vi "Settings IO.vi"(7 "SettingsFileIO_Commands":T2, 8 "Error In":errorcluster, 10 "File Path (for scan specific settings)":path, 11 "Settings Array IN":T1[](array[typedef])) -> (0 "Error Out":errorcluster, 2 "Cancelled?":bool, 3 "Settings Array OUT":T1[](array[typedef]))   [LabVIEW 2012]
doc: "SciScan 1.2 160622"
uses:
  Settings IO_Commands.ctl
  Plugins/Macro Module/MacroGUI Module/Custom Controls and Typedefs/GFG Variable for IO.ctl
panel:
  out "Not found?":bool
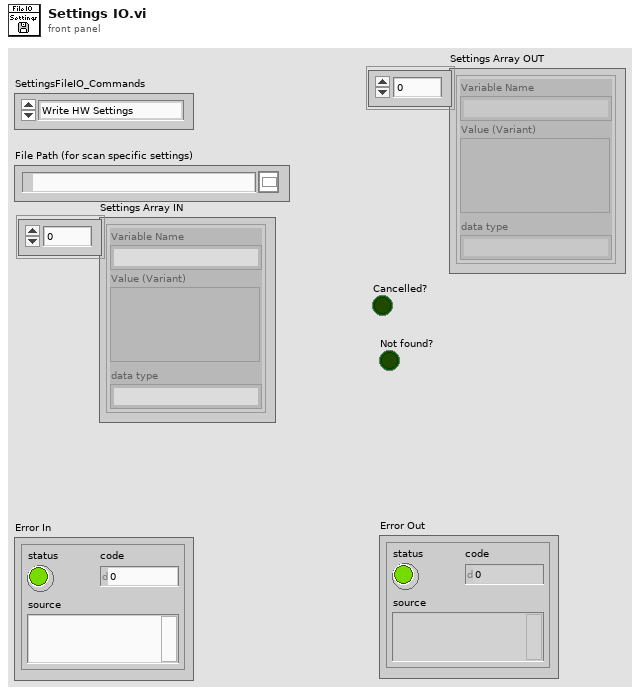
[diagram p1: front panel]
types:
  T1 = typedef "GFG Variable for IO.ctl" = cluster{"Variable Name":string, "Value (Variant)":variant, "data type":string}
  T2 = typedef "Settings IO_Commands.ctl" = enum16{"Write HW Settings", "Write Config Settings", "Read HW Settings", "Read Config Settings", "Write Line-Scan Settings", "Write Frame-Scan Settings", "Write Z-Stack Settings", "Read Line-Scan Settings", "Read Frame-Scan Settings", "Read Z-Stack Settings", "Read Fast-Z Settings", "Write Fast-Z Settings"}
  T3 = typedef "File Operation Status.ctl" = enum16{"Success", "File does not exist", "Cancelled by User", "Incorrect extension type"}
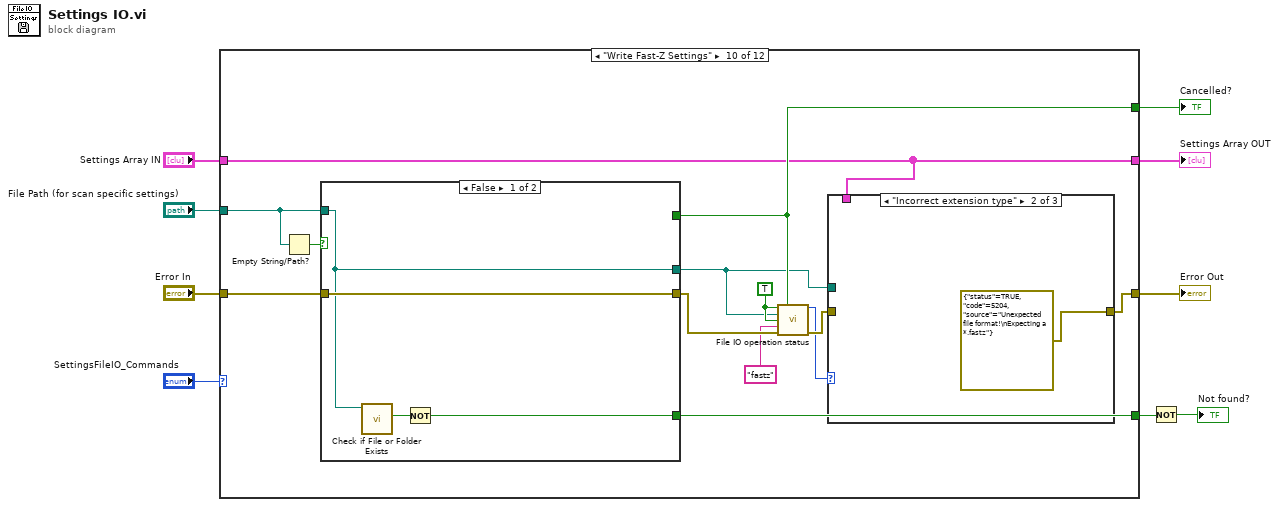
[diagram p0: block diagram]
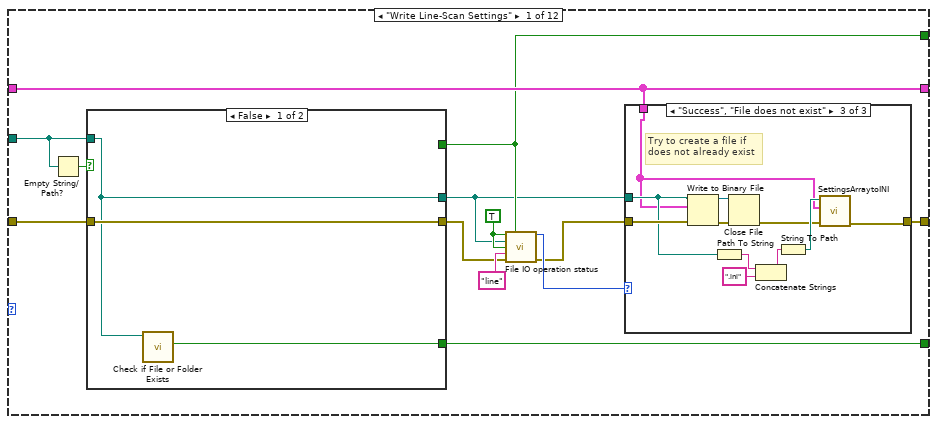
[diagram p2: hidden frame]
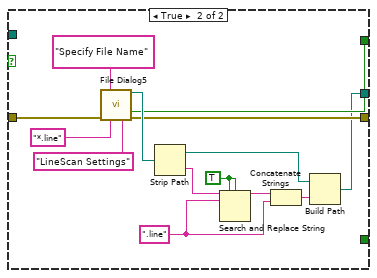
[diagram p3: hidden frame]
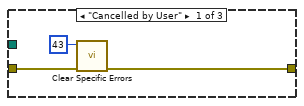
[diagram p4: hidden frame]
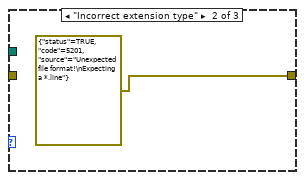
[diagram p5: hidden frame]
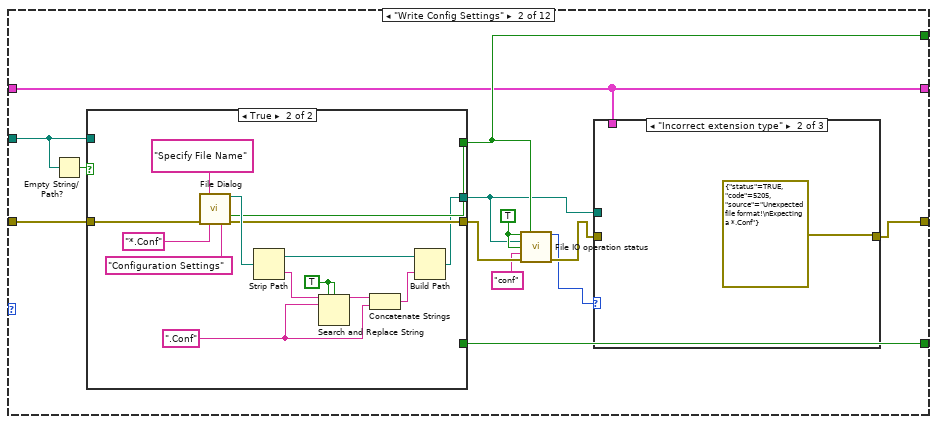
[diagram p6: hidden frame]
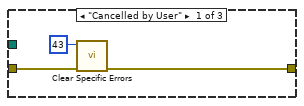
[diagram p7: hidden frame]
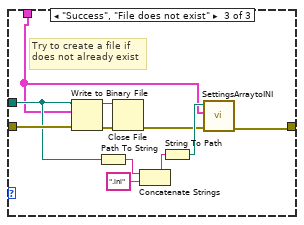
[diagram p8: hidden frame]
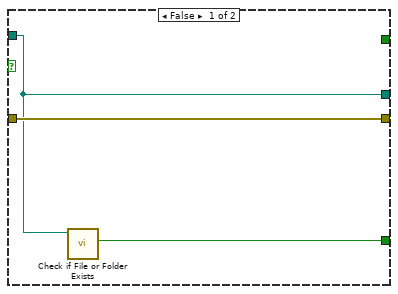
[diagram p9: hidden frame]
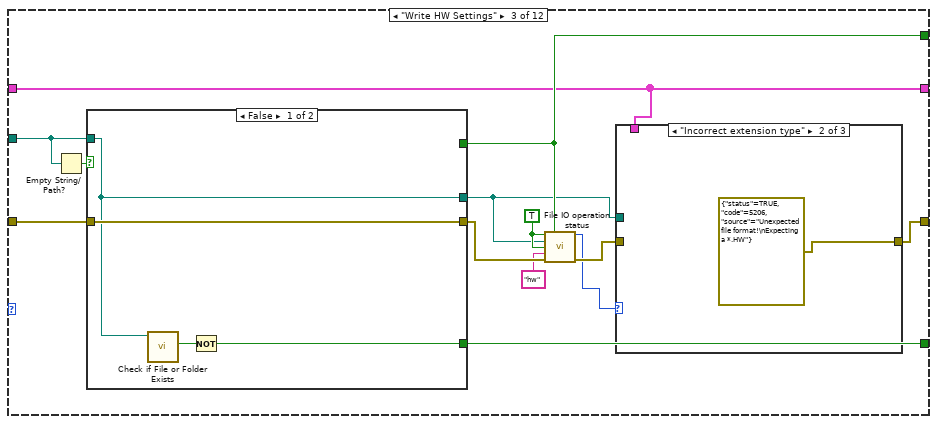
[diagram p10: hidden frame]
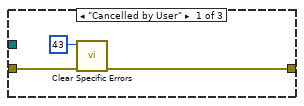
[diagram p11: hidden frame]
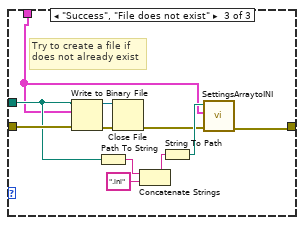
[diagram p12: hidden frame]
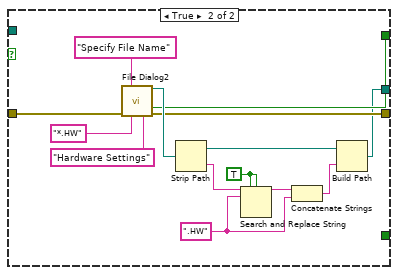
[diagram p13: hidden frame]
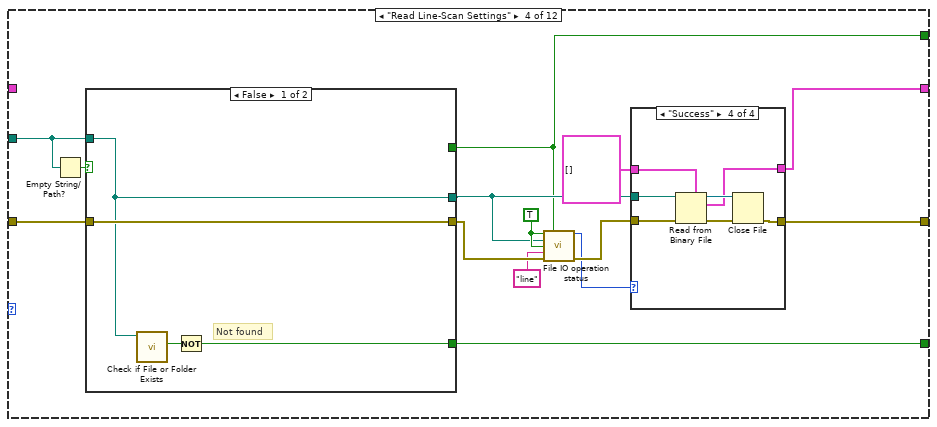
[diagram p14: hidden frame]
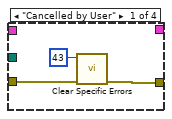
[diagram p15: hidden frame]
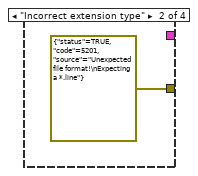
[diagram p16: hidden frame]
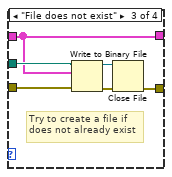
[diagram p17: hidden frame]
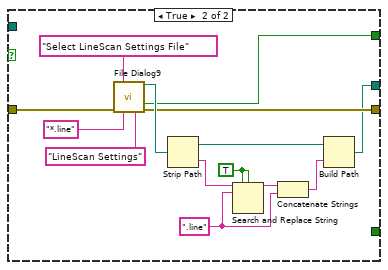
[diagram p18: hidden frame]
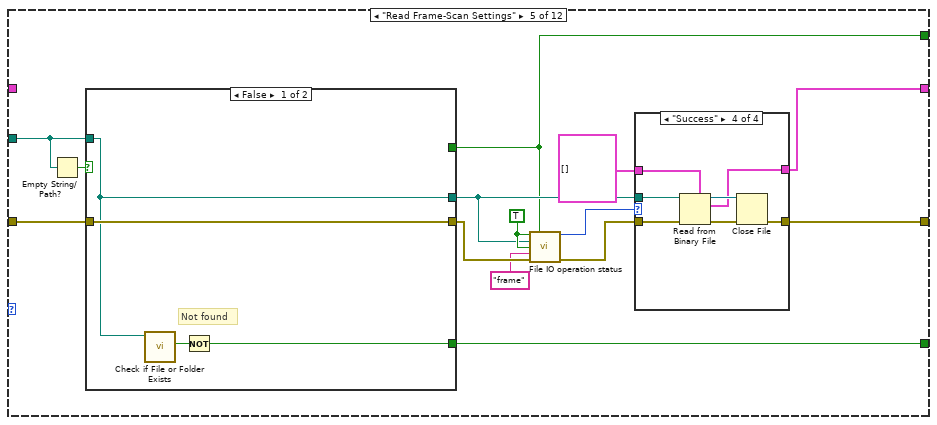
[diagram p19: hidden frame]
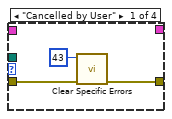
[diagram p20: hidden frame]
diagram:
  n1 = case shown="\"Write Fast-Z Settings\"" "SettingsFileIO_Commands" {
    tunnel: "Settings Array IN" -> [w22 w59 w104 _ _ _ _ w346 w391 w438 _ _]
    tunnel: [w12 w62 w105 w148 w196 w244 w296 w348 w393 w439 w483 w531] -> w7
    tunnel: [w22 w59 w104 w147 w198 w248 w293 w346 w391 w438 w481 w532] -> w6
    tunnel: [w21 w55 w100 w146 w200 w249 w298 w343 w392 w434 w482 w533] -> w5
    tunnel: "Error In" -> [w20 w67 w112 w159 w208 w257 w306 w354 w400 w446 w493 w541]
    tunnel: "File Path (for scan specific settings)" -> [w19 w66 w111 w157 w207 w255 w304 w353 w399 w445 w491 w540]
    tunnel: [w17 w64 w109 w156 w205 w254 w303 w351 w397 w443 w490 w538] -> w2
    frame "Write Line-Scan Settings" {
      w15 = TRUE
      n2 = Empty String/Path?(string/path=w19) -> (empty?=w18:bool)
      n3 = case shown="False" w18 {
        tunnel: [_ w31] -> w12
        tunnel: w20 -> [w25 w28]
        tunnel: [w25 w27] -> w13
        tunnel: w19 -> [w24 _]
        tunnel: [w24 w26] -> w10
        tunnel: [w23 _] -> w17
        frame False {
          n4 = call <vilib>:"Check if File or Folder Exists.vi"("path"=w24) -> ("file or folder exists?"=w23:bool)  [unwired: 8 in, 2 out]
        }
        frame True {
          w32 = ".line" ("pattern (all files)")
          w37 = TRUE ("replace all? (F)")
          n5 = call "File Dialog5"("prompt"="Specify File Name", "error in"=w28, "pattern (all files)"="*.line", "pattern label"="LineScan Settings") -> ("selected path"=w34:path, "cancelled"=w31:bool, "error out"=w27:errorcluster)  [unwired: 8 in, 1 out]
          n6 = Strip Path(path=w34) -> (stripped path=w29:path, name=w36:string)
          n7 = Search and Replace String(replace all?=w37, case sensitive?=w37, input string=w36, search string=w32) -> (result string=w35:string)  [unwired: 4 in, 3 out]
          n8 = Concatenate Strings(w35, w32) -> (w30:string)
          n9 = Build Path(base path=w29, name or relative path=w30) -> (appended path=w26:path)
        }
      }
      n10 = call "File IO operation status.vi"("check if valid path (Specify File Path)"=w15, "Cancelled by User? (status from a previous dialog)"=w12, "File Path"=w10, "check if valid extension (Specify Extension Type)"=w15, "expected extension type"="line" ("string"), "error in (no error)"=w13) -> ("File Operation Status"=w14:T3, "error out"=w11:errorcluster)  [unwired: 8 in]
      n11 = case shown="\"Success\", \"File does not exist\"" w14 {
        tunnel: w22 -> [_ _ w44]
        tunnel: [w40 errorcluster {"status"=TRUE, "code"=5201, "source"="Unexpected file format!\nExpecting a *.line"} ("error constant") w47] -> w21
        tunnel: w11 -> [w41 _ w52]
        tunnel: w10 -> [_ _ w45]
        frame "Cancelled by User" {
          n12 = call "Clear Specific Errors.vi"("Error In"=w41, "Error number In"=43) -> ("Error Out"=w40:errorcluster)  [unwired: 8 in, 1 out]
        }
        frame "Incorrect extension type" {
        }
        frame "Success", "File does not exist" {
          # "Try to create a file if \ndoes not already exist"
          n13 = Write to Binary File(file (use dialog)=w45, data=w44, error in=w52) -> (refnum out=w54:refnum<file>, error out=w53:errorcluster)  [unwired: 3 in, 1 out]
          n14 = Path To String(path=w45) -> (string=w48:string)
          n15 = Close File(refnum=w54, error in=w53) -> (error out=w46:errorcluster)  [unwired: 1 out]
          n16 = Concatenate Strings(w48, ".ini" ("string")) -> (w50:string)
          n17 = String To Path(string=w50) -> (path=w51:path)
          n18 = call "SettingsArraytoINI.vi"("error in (no error)"=w46, "Settings Array IN"=w44, "Path"=w51) -> ("error out"=w47:errorcluster)  [unwired: 8 in]
        }
      }
    }
    frame "Write Config Settings" {
      w63 = TRUE
      n19 = Empty String/Path?(string/path=w66) -> (empty?=w65:bool)
      n20 = case shown="True" w65 {
        tunnel: [_ w91] -> w62
        tunnel: w67 -> [w85 w88]
        tunnel: [w85 w87] -> w61
        tunnel: w66 -> [w84 _]
        tunnel: [w84 w86] -> w58
        tunnel: [w83 _] -> w64
        frame False {
          n21 = call <vilib>:"Check if File or Folder Exists.vi"("path"=w84) -> ("file or folder exists?"=w83:bool)  [unwired: 8 in, 2 out]
        }
        frame True {
          w92 = ".Conf" ("pattern (all files)")
          w97 = TRUE ("replace all? (F)")
          n22 = call "File Dialog"("prompt"="Specify File Name", "error in"=w88, "pattern (all files)"="*.Conf", "pattern label"="Configuration Settings") -> ("selected path"=w94:path, "cancelled"=w91:bool, "error out"=w87:errorcluster)  [unwired: 8 in, 1 out]
          n23 = Strip Path(path=w94) -> (stripped path=w89:path, name=w96:string)
          n24 = Search and Replace String(replace all?=w97, case sensitive?=w97, input string=w96, search string=w92) -> (result string=w95:string)  [unwired: 4 in, 3 out]
          n25 = Concatenate Strings(w95, w92) -> (w90:string)
          n26 = Build Path(base path=w89, name or relative path=w90) -> (appended path=w86:path)
        }
      }
      n27 = call "File IO operation status.vi"("check if valid path (Specify File Path)"=w63, "Cancelled by User? (status from a previous dialog)"=w62, "File Path"=w58, "check if valid extension (Specify Extension Type)"=w63, "expected extension type"="conf" ("string"), "error in (no error)"=w61) -> ("File Operation Status"=w56:T3, "error out"=w57:errorcluster)  [unwired: 8 in]
      n28 = case shown="\"Incorrect extension type\"" w56 {
        tunnel: w59 -> [_ _ w72]
        tunnel: [w68 errorcluster {"status"=TRUE, "code"=5205, "source"="Unexpected file format!\nExpecting a *.Conf"} ("error constant") w75] -> w55
        tunnel: w57 -> [w69 _ w80]
        tunnel: w58 -> [_ _ w73]
        frame "Cancelled by User" {
          n29 = call "Clear Specific Errors.vi"("Error In"=w69, "Error number In"=43) -> ("Error Out"=w68:errorcluster)  [unwired: 8 in, 1 out]
        }
        frame "Incorrect extension type" {
        }
        frame "Success", "File does not exist" {
          # "Try to create a file if \ndoes not already exist"
          n30 = Write to Binary File(file (use dialog)=w73, data=w72, error in=w80) -> (refnum out=w82:refnum<file>, error out=w81:errorcluster)  [unwired: 3 in, 1 out]
          n31 = Path To String(path=w73) -> (string=w76:string)
          n32 = Close File(refnum=w82, error in=w81) -> (error out=w74:errorcluster)  [unwired: 1 out]
          n33 = Concatenate Strings(w76, ".ini" ("string")) -> (w78:string)
          n34 = String To Path(string=w78) -> (path=w79:path)
          n35 = call "SettingsArraytoINI.vi"("error in (no error)"=w74, "Settings Array IN"=w72, "Path"=w79) -> ("error out"=w75:errorcluster)  [unwired: 8 in]
        }
      }
    }
    frame "Write HW Settings" {
      w108 = TRUE
      n36 = Empty String/Path?(string/path=w111) -> (empty?=w110:bool)
      n37 = case shown="False" w110 {
        tunnel: [_ w137] -> w105
        tunnel: w112 -> [w131 w134]
        tunnel: [w131 w133] -> w107
        tunnel: w111 -> [w129 _]
        tunnel: [w129 w132] -> w103
        tunnel: [w128 _] -> w109
        frame False {
          n38 = call <vilib>:"Check if File or Folder Exists.vi"("path"=w129) -> ("file or folder exists?"=w130:bool)  [unwired: 8 in, 2 out]
          n39 = Not(x=w130) -> (.not. x?=w128:bool)
        }
        frame True {
          w138 = ".HW" ("pattern (all files)")
          w143 = TRUE ("replace all? (F)")
          n40 = call "File Dialog2"("prompt"="Specify File Name", "error in"=w134, "pattern (all files)"="*.HW", "pattern label"="Hardware Settings") -> ("selected path"=w140:path, "cancelled"=w137:bool, "error out"=w133:errorcluster)  [unwired: 8 in, 1 out]
          n41 = Strip Path(path=w140) -> (stripped path=w135:path, name=w142:string)
          n42 = Search and Replace String(replace all?=w143, case sensitive?=w143, input string=w142, search string=w138) -> (result string=w141:string)  [unwired: 4 in, 3 out]
          n43 = Concatenate Strings(w141, w138) -> (w136:string)
          n44 = Build Path(base path=w135, name or relative path=w136) -> (appended path=w132:path)
        }
      }
      n45 = call "File IO operation status.vi"("check if valid path (Specify File Path)"=w108, "Cancelled by User? (status from a previous dialog)"=w105, "File Path"=w103, "check if valid extension (Specify Extension Type)"=w108, "expected extension type"="hw" ("string"), "error in (no error)"=w107) -> ("File Operation Status"=w101:T3, "error out"=w102:errorcluster)  [unwired: 8 in]
      n46 = case shown="\"Incorrect extension type\"" w101 {
        tunnel: w104 -> [_ _ w117]
        tunnel: [w113 errorcluster {"status"=TRUE, "code"=5206, "source"="Unexpected file format!\nExpecting a *.HW"} ("error constant") w120] -> w100
        tunnel: w102 -> [w114 _ w125]
        tunnel: w103 -> [_ _ w118]
        frame "Cancelled by User" {
          n47 = call "Clear Specific Errors.vi"("Error In"=w114, "Error number In"=43) -> ("Error Out"=w113:errorcluster)  [unwired: 8 in, 1 out]
        }
        frame "Incorrect extension type" {
        }
        frame "Success", "File does not exist" {
          # "Try to create a file if \ndoes not already exist"
          n48 = Write to Binary File(file (use dialog)=w118, data=w117, error in=w125) -> (refnum out=w127:refnum<file>, error out=w126:errorcluster)  [unwired: 3 in, 1 out]
          n49 = Path To String(path=w118) -> (string=w121:string)
          n50 = Close File(refnum=w127, error in=w126) -> (error out=w119:errorcluster)  [unwired: 1 out]
          n51 = Concatenate Strings(w121, ".ini" ("string")) -> (w123:string)
          n52 = String To Path(string=w123) -> (path=w124:path)
          n53 = call "SettingsArraytoINI.vi"("error in (no error)"=w119, "Settings Array IN"=w117, "Path"=w124) -> ("error out"=w120:errorcluster)  [unwired: 8 in]
        }
      }
    }
    frame "Read Line-Scan Settings" {
      w152 = TRUE
      n54 = Empty String/Path?(string/path=w157) -> (empty?=w158:bool)
      n55 = case shown="False" w158 {
        tunnel: w159 -> [w180 w184]
        tunnel: [w180 w183] -> w151
        tunnel: [w178 w182] -> w149
        tunnel: [_ w181] -> w148
        tunnel: w157 -> [w178 _]
        tunnel: [w177 _] -> w156
        frame False {
          # "Not found"
          n56 = call <vilib>:"Check if File or Folder Exists.vi"("path"=w178) -> ("file or folder exists?"=w179:bool)  [unwired: 8 in, 2 out]
          n57 = Not(x=w179) -> (.not. x?=w177:bool)
        }
        frame True {
          w185 = ".line" ("pattern (all files)")
          w192 = TRUE ("replace all? (F)")
          n58 = call "File Dialog9"("prompt"="Select LineScan Settings File", "error in"=w184, "pattern (all files)"="*.line", "pattern label"="LineScan Settings") -> ("selected path"=w187:path, "cancelled"=w181:bool, "error out"=w183:errorcluster)  [unwired: 8 in, 1 out]
          n59 = Strip Path(path=w187) -> (stripped path=w189:path, name=w191:string)
          n60 = Search and Replace String(replace all?=w192, case sensitive?=w192, input string=w191, search string=w185) -> (result string=w190:string)  [unwired: 4 in, 3 out]
          n61 = Concatenate Strings(w190, w185) -> (w188:string)
          n62 = Build Path(base path=w189, name or relative path=w188) -> (appended path=w182:path)
        }
      }
      n63 = call "File IO operation status.vi"("check if valid path (Specify File Path)"=w152, "Cancelled by User? (status from a previous dialog)"=w148, "File Path"=w149, "check if valid extension (Specify Extension Type)"=w152, "expected extension type"="line" ("string"), "error in (no error)"=w151) -> ("File Operation Status"=w153:T3, "error out"=w154:errorcluster)  [unwired: 8 in]
      n64 = case shown="\"Success\"" w153 {
        tunnel: T1[] [] ("Settings Array IN") -> [_ _ w164 w172]
        tunnel: [w160 errorcluster {"status"=TRUE, "code"=5201, "source"="Unexpected file format!\nExpecting a *.line"} ("error constant") w166 w173] -> w146
        tunnel: w154 -> [w161 _ w167 w174]
        tunnel: w149 -> [_ _ w165 w170]
        tunnel: [_ _ w164 w171] -> w147
        frame "Cancelled by User" {
          n65 = call "Clear Specific Errors.vi"("Error In"=w161, "Error number In"=43) -> ("Error Out"=w160:errorcluster)  [unwired: 8 in, 1 out]
        }
        frame "Incorrect extension type" {
        }
        frame "File does not exist" {
          # "Try to create a file if \ndoes not already exist"
          n66 = Write to Binary File(file (use dialog)=w165, data=w164, error in=w167) -> (refnum out=w169:refnum<file>, error out=w168:errorcluster)  [unwired: 3 in, 1 out]
          n67 = Close File(refnum=w169, error in=w168) -> (error out=w166:errorcluster)  [unwired: 1 out]
        }
        frame "Success" {
          n68 = Read from Binary File(5:w172, 8:w174, 11:w170) -> (0:w176:errorcluster, 2:w171:T1[], 3:w175:refnum<file>)  [unwired: 3 in, 1 out]
          n69 = Close File(refnum=w175, error in=w176) -> (error out=w173:errorcluster)  [unwired: 1 out]
        }
      }
    }
    frame "Read Frame-Scan Settings" {
      w201 = TRUE
      n70 = Empty String/Path?(string/path=w207) -> (empty?=w206:bool)
      n71 = case shown="False" w206 {
        tunnel: w208 -> [w229 w233]
        tunnel: [w229 w232] -> w199
        tunnel: [w227 w231] -> w197
        tunnel: [_ w230] -> w196
        tunnel: w207 -> [w227 _]
        tunnel: [w226 _] -> w205
        frame False {
          # "Not found"
          n72 = call <vilib>:"Check if File or Folder Exists.vi"("path"=w227) -> ("file or folder exists?"=w228:bool)  [unwired: 8 in, 2 out]
          n73 = Not(x=w228) -> (.not. x?=w226:bool)
        }
        frame True {
          w234 = ".frame" ("pattern (all files)")
          w241 = TRUE ("replace all? (F)")
          n74 = call "File Dialog10"("prompt"="Select FrameScan Settings File", "error in"=w233, "pattern (all files)"="*.frame", "pattern label"="FrameScan Settings") -> ("selected path"=w236:path, "cancelled"=w230:bool, "error out"=w232:errorcluster)  [unwired: 8 in, 1 out]
          n75 = Strip Path(path=w236) -> (stripped path=w238:path, name=w240:string)
          n76 = Search and Replace String(replace all?=w241, case sensitive?=w241, input string=w240, search string=w234) -> (result string=w239:string)  [unwired: 4 in, 3 out]
          n77 = Concatenate Strings(w239, w234) -> (w237:string)
          n78 = Build Path(base path=w238, name or relative path=w237) -> (appended path=w231:path)
        }
      }
      n79 = call "File IO operation status.vi"("check if valid path (Specify File Path)"=w201, "Cancelled by User? (status from a previous dialog)"=w196, "File Path"=w197, "check if valid extension (Specify Extension Type)"=w201, "expected extension type"="frame" ("string"), "error in (no error)"=w199) -> ("File Operation Status"=w202:T3, "error out"=w203:errorcluster)  [unwired: 8 in]
      n80 = case shown="\"Success\"" w202 {
        tunnel: T1[] [] ("Settings Array IN") -> [_ _ w213 w221]
        tunnel: [w209 errorcluster {"status"=TRUE, "code"=5202, "source"="Unexpected file format!\nExpecting a *.frame"} ("error constant") w215 w222] -> w200
        tunnel: w203 -> [w210 _ w216 w223]
        tunnel: w197 -> [_ _ w214 w219]
        tunnel: [_ _ w213 w220] -> w198
        frame "Cancelled by User" {
          n81 = call "Clear Specific Errors.vi"("Error In"=w210, "Error number In"=43) -> ("Error Out"=w209:errorcluster)  [unwired: 8 in, 1 out]
        }
        frame "Incorrect extension type" {
        }
        frame "File does not exist" {
          # "Try to create a file if \ndoes not already exist"
          n82 = Write to Binary File(file (use dialog)=w214, data=w213, error in=w216) -> (refnum out=w218:refnum<file>, error out=w217:errorcluster)  [unwired: 3 in, 1 out]
          n83 = Close File(refnum=w218, error in=w217) -> (error out=w215:errorcluster)  [unwired: 1 out]
        }
        frame "Success" {
          n84 = Read from Binary File(5:w221, 8:w223, 11:w219) -> (0:w225:errorcluster, 2:w220:T1[], 3:w224:refnum<file>)  [unwired: 3 in, 1 out]
          n85 = Close File(refnum=w224, error in=w225) -> (error out=w222:errorcluster)  [unwired: 1 out]
        }
      }
    }
    frame "Read Z-Stack Settings" {
      w250 = TRUE
      n86 = Empty String/Path?(string/path=w255) -> (empty?=w256:bool)
      n87 = case shown="True" w256 {
        tunnel: w257 -> [w278 w282]
        tunnel: [w278 w281] -> w247
        tunnel: [w276 w280] -> w246
        tunnel: [_ w279] -> w244
        tunnel: w255 -> [w276 _]
        tunnel: [w275 _] -> w254
        frame False {
          # "Not found"
          n88 = call <vilib>:"Check if File or Folder Exists.vi"("path"=w276) -> ("file or folder exists?"=w277:bool)  [unwired: 8 in, 2 out]
          n89 = Not(x=w277) -> (.not. x?=w275:bool)
        }
        frame True {
          w283 = ".zstack" ("pattern (all files)")
          w290 = TRUE ("replace all? (F)")
          n90 = call "File Dialog11"("prompt"="Select ZStack Settings File", "error in"=w282, "pattern (all files)"="*.zstack", "pattern label"="Z-Stack Settings") -> ("selected path"=w285:path, "cancelled"=w279:bool, "error out"=w281:errorcluster)  [unwired: 8 in, 1 out]
          n91 = Strip Path(path=w285) -> (stripped path=w287:path, name=w289:string)
          n92 = Search and Replace String(replace all?=w290, case sensitive?=w290, input string=w289, search string=w283) -> (result string=w288:string)  [unwired: 4 in, 3 out]
          n93 = Concatenate Strings(w288, w283) -> (w286:string)
          n94 = Build Path(base path=w287, name or relative path=w286) -> (appended path=w280:path)
        }
      }
      n95 = call "File IO operation status.vi"("check if valid path (Specify File Path)"=w250, "Cancelled by User? (status from a previous dialog)"=w244, "File Path"=w246, "check if valid extension (Specify Extension Type)"=w250, "expected extension type"="zstack" ("string"), "error in (no error)"=w247) -> ("File Operation Status"=w251:T3, "error out"=w252:errorcluster)  [unwired: 8 in]
      n96 = case shown="\"File does not exist\"" w251 {
        tunnel: T1[] [] ("Settings Array IN") -> [_ _ w262 w271]
        tunnel: [w258 errorcluster {"status"=TRUE, "code"=5203, "source"="Unexpected file format!\nExpecting a *.zstack"} ("error constant") w264 w268] -> w249
        tunnel: w252 -> [w259 _ w265 w272]
        tunnel: w246 -> [_ _ w263 w269]
        tunnel: [_ _ w262 w270] -> w248
        frame "Cancelled by User" {
          n97 = call "Clear Specific Errors.vi"("Error In"=w259, "Error number In"=43) -> ("Error Out"=w258:errorcluster)  [unwired: 8 in, 1 out]
        }
        frame "Incorrect extension type" {
        }
        frame "File does not exist" {
          # "Try to create a file if \ndoes not already exist"
          n98 = Write to Binary File(file (use dialog)=w263, data=w262, error in=w265) -> (refnum out=w267:refnum<file>, error out=w266:errorcluster)  [unwired: 3 in, 1 out]
          n99 = Close File(refnum=w267, error in=w266) -> (error out=w264:errorcluster)  [unwired: 1 out]
        }
        frame "Success" {
          n100 = Read from Binary File(5:w271, 8:w272, 11:w269) -> (0:w274:errorcluster, 2:w270:T1[], 3:w273:refnum<file>)  [unwired: 3 in, 1 out]
          n101 = Close File(refnum=w273, error in=w274) -> (error out=w268:errorcluster)  [unwired: 1 out]
        }
      }
    }
    frame "Read Fast-Z Settings" {
      w299 = TRUE
      n102 = Empty String/Path?(string/path=w304) -> (empty?=w305:bool)
      n103 = case shown="False" w305 {
        tunnel: w306 -> [w327 w331]
        tunnel: [w327 w330] -> w297
        tunnel: [w325 w329] -> w295
        tunnel: [_ w328] -> w296
        tunnel: w304 -> [w325 _]
        tunnel: [w324 _] -> w303
        frame False {
          # "Not found"
          n104 = call <vilib>:"Check if File or Folder Exists.vi"("path"=w325) -> ("file or folder exists?"=w326:bool)  [unwired: 8 in, 2 out]
          n105 = Not(x=w326) -> (.not. x?=w324:bool)
        }
        frame True {
          w332 = ".fastz" ("pattern (all files)")
          w339 = TRUE ("replace all? (F)")
          n106 = call "File Dialog6"("prompt"="Select Fast-Z Settings File", "error in"=w331, "pattern (all files)"="*.fastz", "pattern label"="Fast-Z Settings") -> ("selected path"=w334:path, "cancelled"=w328:bool, "error out"=w330:errorcluster)  [unwired: 8 in, 1 out]
          n107 = Strip Path(path=w334) -> (stripped path=w336:path, name=w338:string)
          n108 = Search and Replace String(replace all?=w339, case sensitive?=w339, input string=w338, search string=w332) -> (result string=w337:string)  [unwired: 4 in, 3 out]
          n109 = Concatenate Strings(w337, w332) -> (w335:string)
          n110 = Build Path(base path=w336, name or relative path=w335) -> (appended path=w329:path)
        }
      }
      n111 = call "File IO operation status.vi"("check if valid path (Specify File Path)"=w299, "Cancelled by User? (status from a previous dialog)"=w296, "File Path"=w295, "check if valid extension (Specify Extension Type)"=w299, "expected extension type"="fastz" ("string"), "error in (no error)"=w297) -> ("File Operation Status"=w300:T3, "error out"=w301:errorcluster)  [unwired: 8 in]
      n112 = case shown="\"Success\"" w300 {
        tunnel: T1[] [] ("Settings Array IN") -> [_ _ w311 w319]
        tunnel: [w307 errorcluster {"status"=TRUE, "code"=5204, "source"="Unexpected file format!\nExpecting a *.fastz"} ("error constant") w313 w320] -> w298
        tunnel: w301 -> [w308 _ w314 w321]
        tunnel: w295 -> [_ _ w312 w317]
        tunnel: [_ _ w311 w318] -> w293
        frame "Cancelled by User" {
          n113 = call "Clear Specific Errors.vi"("Error In"=w308, "Error number In"=43) -> ("Error Out"=w307:errorcluster)  [unwired: 8 in, 1 out]
        }
        frame "Incorrect extension type" {
        }
        frame "File does not exist" {
          # "Try to create a file if \ndoes not already exist"
          n114 = Write to Binary File(file (use dialog)=w312, data=w311, error in=w314) -> (refnum out=w316:refnum<file>, error out=w315:errorcluster)  [unwired: 3 in, 1 out]
          n115 = Close File(refnum=w316, error in=w315) -> (error out=w313:errorcluster)  [unwired: 1 out]
        }
        frame "Success" {
          n116 = Read from Binary File(5:w319, 8:w321, 11:w317) -> (0:w323:errorcluster, 2:w318:T1[], 3:w322:refnum<file>)  [unwired: 3 in, 1 out]
          n117 = Close File(refnum=w322, error in=w323) -> (error out=w320:errorcluster)  [unwired: 1 out]
        }
      }
    }
    frame "Write Frame-Scan Settings" {
      w350 = TRUE
      n118 = Empty String/Path?(string/path=w353) -> (empty?=w352:bool)
      n119 = case shown="False" w352 {
        tunnel: [_ w379] -> w348
        tunnel: w354 -> [w373 w376]
        tunnel: [w373 w375] -> w349
        tunnel: w353 -> [w371 _]
        tunnel: [w371 w374] -> w344
        tunnel: [w370 _] -> w351
        frame False {
          n120 = call <vilib>:"Check if File or Folder Exists.vi"("path"=w371) -> ("file or folder exists?"=w372:bool)  [unwired: 8 in, 2 out]
          n121 = Not(x=w372) -> (.not. x?=w370:bool)
        }
        frame True {
          w380 = ".frame" ("pattern (all files)")
          w385 = TRUE ("replace all? (F)")
          n122 = call "File Dialog7"("prompt"="Specify File Name", "error in"=w376, "pattern (all files)"="*.frame", "pattern label"="FrameScan Settings") -> ("selected path"=w382:path, "cancelled"=w379:bool, "error out"=w375:errorcluster)  [unwired: 8 in, 1 out]
          n123 = Strip Path(path=w382) -> (stripped path=w377:path, name=w384:string)
          n124 = Search and Replace String(replace all?=w385, case sensitive?=w385, input string=w384, search string=w380) -> (result string=w383:string)  [unwired: 4 in, 3 out]
          n125 = Concatenate Strings(w383, w380) -> (w378:string)
          n126 = Build Path(base path=w377, name or relative path=w378) -> (appended path=w374:path)
        }
      }
      n127 = call "File IO operation status.vi"("check if valid path (Specify File Path)"=w350, "Cancelled by User? (status from a previous dialog)"=w348, "File Path"=w344, "check if valid extension (Specify Extension Type)"=w350, "expected extension type"="frame" ("string"), "error in (no error)"=w349) -> ("File Operation Status"=w342:T3, "error out"=w345:errorcluster)  [unwired: 8 in]
      n128 = case shown="\"Incorrect extension type\"" w342 {
        tunnel: w346 -> [_ _ w359]
        tunnel: [w355 errorcluster {"status"=TRUE, "code"=5202, "source"="Unexpected file format!\nExpecting a *.frame"} ("error constant") w362] -> w343
        tunnel: w345 -> [w356 _ w367]
        tunnel: w344 -> [_ _ w360]
        frame "Cancelled by User" {
          n129 = call "Clear Specific Errors.vi"("Error In"=w356, "Error number In"=43) -> ("Error Out"=w355:errorcluster)  [unwired: 8 in, 1 out]
        }
        frame "Incorrect extension type" {
        }
        frame "Success", "File does not exist" {
          # "Try to create a file if \ndoes not already exist"
          n130 = Write to Binary File(file (use dialog)=w360, data=w359, error in=w367) -> (refnum out=w369:refnum<file>, error out=w368:errorcluster)  [unwired: 3 in, 1 out]
          n131 = Path To String(path=w360) -> (string=w363:string)
          n132 = Close File(refnum=w369, error in=w368) -> (error out=w361:errorcluster)  [unwired: 1 out]
          n133 = Concatenate Strings(w363, ".ini" ("string")) -> (w365:string)
          n134 = String To Path(string=w365) -> (path=w366:path)
          n135 = call "SettingsArraytoINI.vi"("error in (no error)"=w361, "Settings Array IN"=w359, "Path"=w366) -> ("error out"=w362:errorcluster)  [unwired: 8 in]
        }
      }
    }
    frame "Write Z-Stack Settings" {
      w396 = TRUE
      n136 = Empty String/Path?(string/path=w399) -> (empty?=w398:bool)
      n137 = case shown="True" w398 {
        tunnel: [_ w425] -> w393
        tunnel: w400 -> [w419 w422]
        tunnel: [w419 w421] -> w395
        tunnel: w399 -> [w417 _]
        tunnel: [w417 w420] -> w390
        tunnel: [w416 _] -> w397
        frame False {
          n138 = call <vilib>:"Check if File or Folder Exists.vi"("path"=w417) -> ("file or folder exists?"=w418:bool)  [unwired: 8 in, 2 out]
          n139 = Not(x=w418) -> (.not. x?=w416:bool)
        }
        frame True {
          w426 = ".zstack" ("pattern (all files)")
          w431 = TRUE ("replace all? (F)")
          n140 = call "File Dialog8"("prompt"="Specify File Name", "error in"=w422, "pattern (all files)"="*.zstack", "pattern label"="Z-Stack Settings") -> ("selected path"=w428:path, "cancelled"=w425:bool, "error out"=w421:errorcluster)  [unwired: 8 in, 1 out]
          n141 = Strip Path(path=w428) -> (stripped path=w423:path, name=w430:string)
          n142 = Search and Replace String(replace all?=w431, case sensitive?=w431, input string=w430, search string=w426) -> (result string=w429:string)  [unwired: 4 in, 3 out]
          n143 = Concatenate Strings(w429, w426) -> (w424:string)
          n144 = Build Path(base path=w423, name or relative path=w424) -> (appended path=w420:path)
        }
      }
      n145 = call "File IO operation status.vi"("check if valid path (Specify File Path)"=w396, "Cancelled by User? (status from a previous dialog)"=w393, "File Path"=w390, "check if valid extension (Specify Extension Type)"=w396, "expected extension type"="zstack" ("string"), "error in (no error)"=w395) -> ("File Operation Status"=w388:T3, "error out"=w389:errorcluster)  [unwired: 8 in]
      n146 = case shown="\"Incorrect extension type\"" w388 {
        tunnel: w391 -> [_ _ w405]
        tunnel: [w401 errorcluster {"status"=TRUE, "code"=5203, "source"="Unexpected file format!\nExpecting a *.zstack"} ("error constant") w408] -> w392
        tunnel: w389 -> [w402 _ w413]
        tunnel: w390 -> [_ _ w406]
        frame "Cancelled by User" {
          n147 = call "Clear Specific Errors.vi"("Error In"=w402, "Error number In"=43) -> ("Error Out"=w401:errorcluster)  [unwired: 8 in, 1 out]
        }
        frame "Incorrect extension type" {
        }
        frame "Success", "File does not exist" {
          # "Try to create a file if \ndoes not already exist"
          n148 = Write to Binary File(file (use dialog)=w406, data=w405, error in=w413) -> (refnum out=w415:refnum<file>, error out=w414:errorcluster)  [unwired: 3 in, 1 out]
          n149 = Path To String(path=w406) -> (string=w409:string)
          n150 = Close File(refnum=w415, error in=w414) -> (error out=w407:errorcluster)  [unwired: 1 out]
          n151 = Concatenate Strings(w409, ".ini" ("string")) -> (w411:string)
          n152 = String To Path(string=w411) -> (path=w412:path)
          n153 = call "SettingsArraytoINI.vi"("error in (no error)"=w407, "Settings Array IN"=w405, "Path"=w412) -> ("error out"=w408:errorcluster)  [unwired: 8 in]
        }
      }
    }
    frame "Write Fast-Z Settings" {
      w442 = TRUE
      n154 = Empty String/Path?(string/path=w445) -> (empty?=w444:bool)
      n155 = case shown="False" w444 {
        tunnel: [_ w471] -> w439
        tunnel: w446 -> [w465 w468]
        tunnel: [w465 w467] -> w441
        tunnel: w445 -> [w463 _]
        tunnel: [w463 w466] -> w437
        tunnel: [w462 _] -> w443
        frame False {
          n156 = call <vilib>:"Check if File or Folder Exists.vi"("path"=w463) -> ("file or folder exists?"=w464:bool)  [unwired: 8 in, 2 out]
          n157 = Not(x=w464) -> (.not. x?=w462:bool)
        }
        frame True {
          w472 = ".fastz" ("pattern (all files)")
          w477 = TRUE ("replace all? (F)")
          n158 = call "File Dialog12"("prompt"="Specify File Name", "error in"=w468, "pattern (all files)"="*.fastz", "pattern label"="Fast-Z Settings") -> ("selected path"=w474:path, "cancelled"=w471:bool, "error out"=w467:errorcluster)  [unwired: 8 in, 1 out]
          n159 = Strip Path(path=w474) -> (stripped path=w469:path, name=w476:string)
          n160 = Search and Replace String(replace all?=w477, case sensitive?=w477, input string=w476, search string=w472) -> (result string=w475:string)  [unwired: 4 in, 3 out]
          n161 = Concatenate Strings(w475, w472) -> (w470:string)
          n162 = Build Path(base path=w469, name or relative path=w470) -> (appended path=w466:path)
        }
      }
      n163 = call "File IO operation status.vi"("check if valid path (Specify File Path)"=w442, "Cancelled by User? (status from a previous dialog)"=w439, "File Path"=w437, "check if valid extension (Specify Extension Type)"=w442, "expected extension type"="fastz" ("string"), "error in (no error)"=w441) -> ("File Operation Status"=w435:T3, "error out"=w436:errorcluster)  [unwired: 8 in]
      n164 = case shown="\"Incorrect extension type\"" w435 {
        tunnel: w438 -> [_ _ w451]
        tunnel: [w447 errorcluster {"status"=TRUE, "code"=5204, "source"="Unexpected file format!\nExpecting a *.fastz"} ("error constant") w454] -> w434
        tunnel: w436 -> [w448 _ w459]
        tunnel: w437 -> [_ _ w452]
        frame "Cancelled by User" {
          n165 = call "Clear Specific Errors.vi"("Error In"=w448, "Error number In"=43) -> ("Error Out"=w447:errorcluster)  [unwired: 8 in, 1 out]
        }
        frame "Incorrect extension type" {
        }
        frame "Success", "File does not exist" {
          # "Try to create a file if \ndoes not already exist"
          n166 = Write to Binary File(file (use dialog)=w452, data=w451, error in=w459) -> (refnum out=w461:refnum<file>, error out=w460:errorcluster)  [unwired: 3 in, 1 out]
          n167 = Path To String(path=w452) -> (string=w455:string)
          n168 = Close File(refnum=w461, error in=w460) -> (error out=w453:errorcluster)  [unwired: 1 out]
          n169 = Concatenate Strings(w455, ".ini" ("string")) -> (w457:string)
          n170 = String To Path(string=w457) -> (path=w458:path)
          n171 = call "SettingsArraytoINI.vi"("error in (no error)"=w453, "Settings Array IN"=w451, "Path"=w458) -> ("error out"=w454:errorcluster)  [unwired: 8 in]
        }
      }
    }
    frame "Read HW Settings" {
      w486 = TRUE
      n172 = Empty String/Path?(string/path=w491) -> (empty?=w492:bool)
      n173 = case shown="False" w492 {
        tunnel: w493 -> [w513 w517]
        tunnel: [w513 w516] -> w485
        tunnel: [w512 w515] -> w484
        tunnel: [_ w514] -> w483
        tunnel: w491 -> [w512 _]
        tunnel: [w511 _] -> w490
        frame False {
          # "Not found"
          n174 = call <vilib>:"Check if File or Folder Exists.vi"("path"=w512) -> ("file or folder exists?"=w511:bool)  [unwired: 8 in, 2 out]
        }
        frame True {
          w518 = ".HW" ("pattern (all files)")
          w525 = TRUE ("replace all? (F)")
          n175 = call "File Dialog3"("prompt"="Select Hardware Settings File", "error in"=w517, "pattern (all files)"="*.HW", "pattern label"="Hardware Settings") -> ("selected path"=w520:path, "cancelled"=w514:bool, "error out"=w516:errorcluster)  [unwired: 8 in, 1 out]
          n176 = Strip Path(path=w520) -> (stripped path=w522:path, name=w524:string)
          n177 = Search and Replace String(replace all?=w525, case sensitive?=w525, input string=w524, search string=w518) -> (result string=w523:string)  [unwired: 4 in, 3 out]
          n178 = Concatenate Strings(w523, w518) -> (w521:string)
          n179 = Build Path(base path=w522, name or relative path=w521) -> (appended path=w515:path)
        }
      }
      n180 = call "File IO operation status.vi"("check if valid path (Specify File Path)"=w486, "Cancelled by User? (status from a previous dialog)"=w483, "File Path"=w484, "check if valid extension (Specify Extension Type)"=w486, "expected extension type"="hw" ("string"), "error in (no error)"=w485) -> ("File Operation Status"=w487:T3, "error out"=w488:errorcluster)  [unwired: 8 in]
      n181 = case shown="\"Incorrect extension type\"" w487 {
        tunnel: T1[] [] ("Settings Array IN") -> [_ _ w498 w506]
        tunnel: [w494 errorcluster {"status"=TRUE, "code"=5206, "source"="Unexpected file format!\nExpecting a *.HW"} ("error constant") w500 w507] -> w482
        tunnel: w488 -> [w495 _ w501 w508]
        tunnel: w484 -> [_ _ w499 w504]
        tunnel: [_ _ w498 w505] -> w481
        frame "Cancelled by User" {
          n182 = call "Clear Specific Errors.vi"("Error In"=w495, "Error number In"=43) -> ("Error Out"=w494:errorcluster)  [unwired: 8 in, 1 out]
        }
        frame "Incorrect extension type" {
        }
        frame "File does not exist" {
          # "Try to create a file if \ndoes not already exist"
          n183 = Write to Binary File(file (use dialog)=w499, data=w498, error in=w501) -> (refnum out=w503:refnum<file>, error out=w502:errorcluster)  [unwired: 3 in, 1 out]
          n184 = Close File(refnum=w503, error in=w502) -> (error out=w500:errorcluster)  [unwired: 1 out]
        }
        frame "Success" {
          n185 = Read from Binary File(5:w506, 8:w508, 11:w504) -> (0:w510:errorcluster, 2:w505:T1[], 3:w509:refnum<file>)  [unwired: 3 in, 1 out]
          n186 = Close File(refnum=w509, error in=w510) -> (error out=w507:errorcluster)  [unwired: 1 out]
        }
      }
    }
    frame "Read Config Settings" {
      w534 = TRUE
      n187 = Empty String/Path?(string/path=w540) -> (empty?=w539:bool)
      n188 = case shown="False" w539 {
        tunnel: w541 -> [w561 w565]
        tunnel: [w561 w564] -> w529
        tunnel: [w560 w563] -> w530
        tunnel: [_ w562] -> w531
        tunnel: w540 -> [w560 _]
        tunnel: [w559 _] -> w538
        frame False {
          n189 = call <vilib>:"Check if File or Folder Exists.vi"("path"=w560) -> ("file or folder exists?"=w559:bool)  [unwired: 8 in, 2 out]
        }
        frame True {
          w566 = ".Conf" ("pattern (all files)")
          w573 = TRUE ("replace all? (F)")
          n190 = call "File Dialog4"("prompt"="Select Config Settings File", "error in"=w565, "pattern (all files)"="*.Conf", "pattern label"="Configuration Settings") -> ("selected path"=w568:path, "cancelled"=w562:bool, "error out"=w564:errorcluster)  [unwired: 8 in, 1 out]
          n191 = Strip Path(path=w568) -> (stripped path=w570:path, name=w572:string)
          n192 = Search and Replace String(replace all?=w573, case sensitive?=w573, input string=w572, search string=w566) -> (result string=w571:string)  [unwired: 4 in, 3 out]
          n193 = Concatenate Strings(w571, w566) -> (w569:string)
          n194 = Build Path(base path=w570, name or relative path=w569) -> (appended path=w563:path)
        }
      }
      n195 = call "File IO operation status.vi"("check if valid path (Specify File Path)"=w534, "Cancelled by User? (status from a previous dialog)"=w531, "File Path"=w530, "check if valid extension (Specify Extension Type)"=w534, "expected extension type"="conf" ("string"), "error in (no error)"=w529) -> ("File Operation Status"=w535:T3, "error out"=w536:errorcluster)  [unwired: 8 in]
      n196 = case shown="\"Incorrect extension type\"" w535 {
        tunnel: T1[] [] ("Settings Array IN") -> [_ _ w546 w554]
        tunnel: [w542 errorcluster {"status"=TRUE, "code"=5205, "source"="Unexpected file format!\nExpecting a *.Conf"} ("error constant") w548 w555] -> w533
        tunnel: w536 -> [w543 _ w549 w556]
        tunnel: w530 -> [_ _ w547 w552]
        tunnel: [_ _ w546 w553] -> w532
        frame "Cancelled by User" {
          n197 = call "Clear Specific Errors.vi"("Error In"=w543, "Error number In"=43) -> ("Error Out"=w542:errorcluster)  [unwired: 8 in, 1 out]
        }
        frame "Incorrect extension type" {
        }
        frame "File does not exist" {
          # "Try to create a file if \ndoes not already exist"
          n198 = Write to Binary File(file (use dialog)=w547, data=w546, error in=w549) -> (refnum out=w551:refnum<file>, error out=w550:errorcluster)  [unwired: 3 in, 1 out]
          n199 = Close File(refnum=w551, error in=w550) -> (error out=w548:errorcluster)  [unwired: 1 out]
        }
        frame "Success" {
          n200 = Read from Binary File(5:w554, 8:w556, 11:w552) -> (0:w558:errorcluster, 2:w553:T1[], 3:w557:refnum<file>)  [unwired: 3 in, 1 out]
          n201 = Close File(refnum=w557, error in=w558) -> (error out=w555:errorcluster)  [unwired: 1 out]
        }
      }
    }
  }
  "Error Out" <- w5
  "Settings Array OUT" <- w6
  "Cancelled?" <- w7
  n202 = Not(x=w2) -> (.not. x?=→"Not found?":bool)
